vi "Start Task.vi"(8 "error in (no error)":errorcluster, 11 "DAQmx Actor in":refnum<class "DAQmx Actor.lvclass">) -> (0 "error out":errorcluster, 3 "DAQmx Actor out":refnum<class "DAQmx Actor.lvclass">)   [LabVIEW 2024, in "DAQmx Actor.lvlib" / "DAQmx Actor.lvclass"]
uses:
  DAQmx Actor.lvclass
  DAQmx Actor.lvclass/DAQmx Actor.ctl
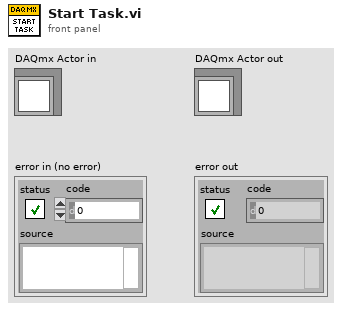
[diagram p1: front panel]
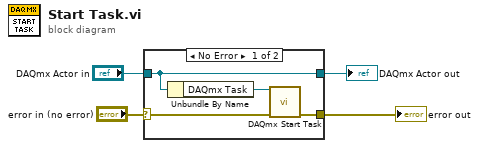
[diagram p0: block diagram]
diagram:
  n1 = case shown="No Error" "error in (no error)" {
    selector: "error in (no error)" -> [w7 w10]
    tunnel: [w6 w10] -> w3
    tunnel: [w5 w9] -> w1
    tunnel: "DAQmx Actor in" -> [w5 w9]
    frame No Error {
      n2 = Unbundle By Name(w5) -> ("DAQmx Task"=w8:refnum<k21>)
      n3 = call <vilib>:"DAQmx Start Task.vi"("task/channels in"=w8, "error in"=w7) -> ("error out"=w6:errorcluster)  [unwired: 12 in, 1 out]
    }
    frame Error {
    }
  }
  "error out" <- w3
  "DAQmx Actor out" <- w1
